vi "switchToStreamMode.vi"(8 "error in (no error)":errorcluster, 9 "Stream Mode Algorithm":T1, 10 "model":refnum<class "Model.lvclass">, 11 "State in":refnum<class "State.lvclass">) -> (0 "error out":errorcluster, 2 "model 2":refnum<class "Model.lvclass">, 3 "State out":refnum<class "State.lvclass">)   [LabVIEW 2013, in "State.lvclass"]
uses:
  State.lvclass
  Model/Model/Model.lvclass
  Configuration/Stream Mode Algorithm.ctl
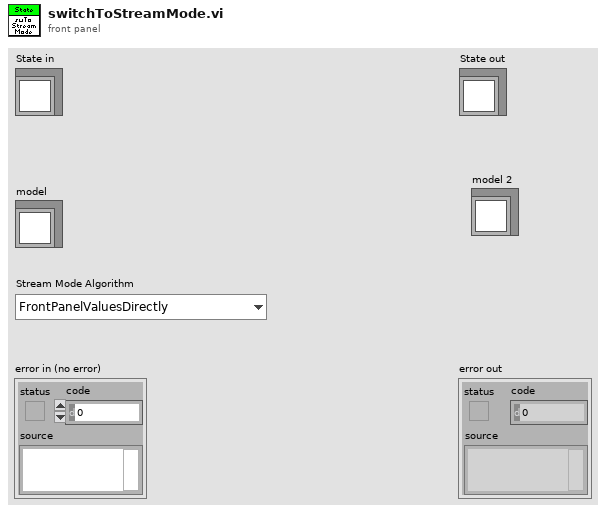
[diagram p1: front panel]
types:
  T1 = typedef "Stream Mode Algorithm.ctl" = enum16{"FrontPanelValuesDirectly"}
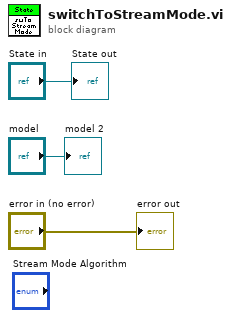
[diagram p0: block diagram]
diagram:
  "error out" <- "error in (no error)"
  "State out" <- "State in"
  "model 2" <- "model"
